vi "HexToString.vi"(10 "字符个数":i32=6, 11 "数组":u16[](array[numeric]) format="%04xH") -> (3 "STRING":string[](array[string]))   [LabVIEW 2016, in "质控单元V2.lvlib"]
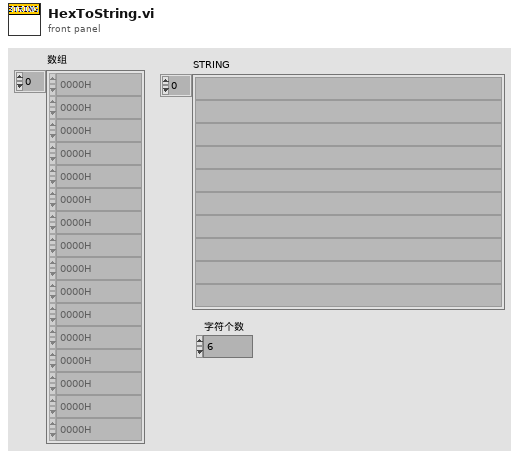
[diagram p1: front panel]
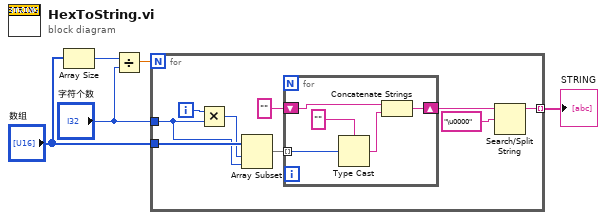
[diagram p0: block diagram]
diagram:
  n1 = Array Size(array="数组") -> (size(s)=w5:i32)
  n2 = Divide(x=w5, y="字符个数") -> (x/y=w4:dbl)
  n3 = for {
    N: w4 -> [_]
    tunnel: "数组" -> [w14]
    tunnel: [w8] -> w3 mode=indexing
    tunnel: "字符个数" -> [w7]
    i -> [w13]
    n4 = Multiply(x=w13, y=w7) -> (x*y=w12:i32)
    n5 = Array Subset(array=w14, index=w12, length=w7) -> (w10:u16[])
    n6 = for {
      shift-right: [w19] -> w9
      shift-left: "" -> [w16]
      tunnel: w10 -> [w18] mode=indexing
      n7 = Type Cast(type="", x=w18) -> (*(type *) &x=w15:string)
      n8 = Concatenate Strings(w16, w15) -> (w19:string)
    }
    n9 = Search/Split String(string=w9, search string/char (-)="\u0000" ("搜索字符串")) -> (substring before match=w8:string)  [unwired: 1 in, 2 out]
  }
  "STRING" <- w3
